vi "Connect to Slave.vi"(8 "error in (no error)":errorcluster, 11 "network master in":refnum<class "WebSocket Client CR.lvclass">) -> (0 "error out":errorcluster, 3 "network master out":refnum<class "WebSocket Client CR.lvclass">)   [LabVIEW 2021, in "WebSockets.lvlib" / "WebSocket Client CR.lvclass"]
doc: "This provides an interface for the master to open a connection to the slave."
uses:
  WebSocket Client CR.lvclass
  WebSocket Client CR.lvclass/WebSocket Client CR.ctl
  WebSocket/WebSocket.lvclass/WebSocket.ctl
  Sockets/Socket/Socket.lvclass
  WebSocket/WebSocket.lvclass
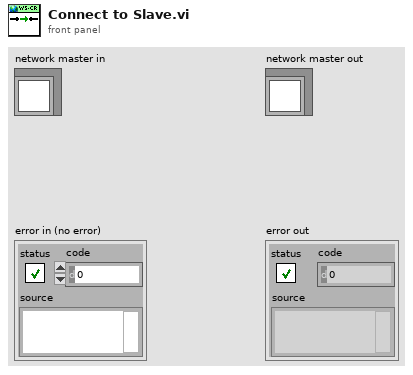
[diagram p1: front panel]
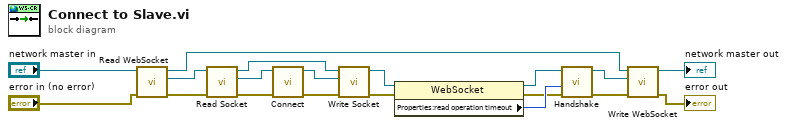
[diagram p0: block diagram]
diagram:
  n1 = call "Read WebSocket.vi"("error in (no error)"="error in (no error)", "Master CR in"="network master in") -> ("error out"=w17:errorcluster, "WebSocket"=w18:refnum<class "WebSocket.lvclass">, "Master CR out"=w11:refnum<class "WebSocket Client CR.lvclass">)  [unwired: 7 in]
  n2 = call "Read Socket.vi"("error in (no error)"=w17, "WebSocket in"=w18) -> ("error out"=w15:errorcluster, "Socket"=w16:refnum<class "Socket.lvclass">, "WebSocket out"=w12:refnum<class "WebSocket.lvclass">)  [unwired: 7 in]
  n3 = call-dynamic "Connect.vi"("error in (no error)"=w15, "Socket in"=w16) -> ("error out"=w14:errorcluster, "Socket out"=w13:refnum<class "Socket.lvclass">)  [unwired: 8 in]
  n4 = call "Write Socket.vi"("error in (no error)"=w14, "Socket"=w13, "WebSocket in"=w12) -> ("error out"=w4:errorcluster, "WebSocket out"=w5:refnum<class "WebSocket.lvclass">)  [unwired: 7 in]
  n5 = property class="WebSocket"(reference=w5, error in=w4) -> (reference out=w2:refnum<class "WebSocket.lvclass">, error out=w3:errorcluster, "Properties:read operation timeout"=w8:i32)
  n6 = call-dynamic "Handshake.vi"("error in (no error)"=w3, "timeout ms (5000)"=w8, "WebSockets in"=w2) -> ("error out"=w7:errorcluster, "WebSockets out"=w6:refnum<class "WebSocket.lvclass">)  [unwired: 7 in]
  n7 = call "Write WebSocket.vi"("error in (no error)"=w7, "WebSocket"=w6, "Master CR in"=w11) -> ("error out"=→"error out":errorcluster, "Master CR out"=→"network master out":refnum<class "WebSocket Client CR.lvclass">)  [unwired: 7 in]
